vi "CreatePrivateEvents.vi"(8 "error in (no error)":errorcluster, 11 "SMO.Instrument":refnum<class "SMO.Instrument.lvclass">) -> (0 "error out":errorcluster, 3 "SMO.Instrument out":refnum<class "SMO.Instrument.lvclass">)   [LabVIEW 2019, in "SMO.Instrument.lvclass"]
doc: "JKI State Machine Objects (SMO) 1.1.0.20\nJKI - JKI\nCopyright (c) 2016, JKI"
uses:
  SMO.Instrument.lvclass
  SMO.Instrument.lvclass/SMO.Instrument.ctl
  Typedefs/API Inputs--Cluster.ctl
  Typedefs/Data.ctl
  vi.lib/JKI/JKI SMO/SMO/SMO.lvclass
panel:
  # "For instructions on how to use the JKI State Machine Objects, examples and video tutorials, visit:\nhttp://jki.net/state-machine-objects/\n\nJKI State Machine Objects™\nhttp://jki.net/state-machine-objects/\nCopyright (C) 2005-2015, JKI <info@jki.net>\nALL RIGHTS RESERVED"
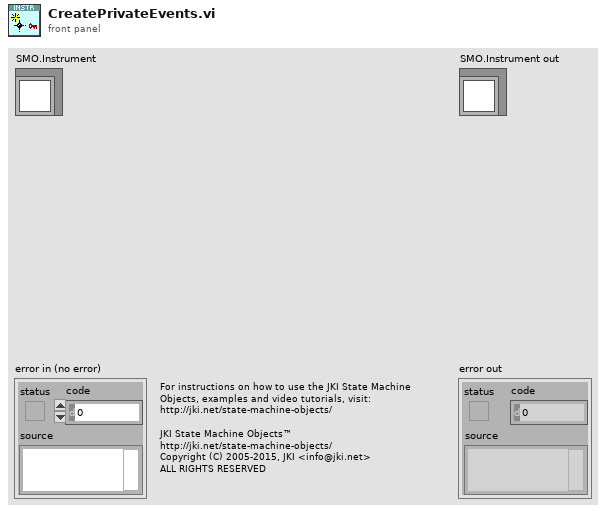
[diagram p1: front panel]
types:
  T1 = typedef "SMO.Instrument.lvclass/PrivateData--Ref.ctl" = refnum<data-value>
  T2 = typedef "SMO.Instrument.lvclass/API Inputs--Cluster.ctl" = cluster{"Data":T3}
  T3 = typedef "SMO.Instrument.lvclass/Data.ctl" = string
  T4 = typedef "SMO.Instrument.lvclass/PrivateData--Cluster.ctl" = cluster{"Configuration":T5, "Public Events":T6, "Protected Events":T7, "Private Events":T8, "Data":T3}
  T5 = typedef "SMO.Instrument.lvclass/Configuration--Cluster.ctl" = cluster{"Suffix":string}
  T6 = typedef "SMO.Instrument.lvclass/PublicEvents--Cluster.ctl" = cluster{"Data Changed":refnum<user-event>}
  T7 = typedef "SMO.Instrument.lvclass/ProtectedEvents--Cluster.ctl" = cluster{"API_Template":refnum<user-event>}
  T8 = typedef "SMO.Instrument.lvclass/PrivateEvents--Cluster.ctl" = cluster{"AsyncMethod":refnum<user-event>}
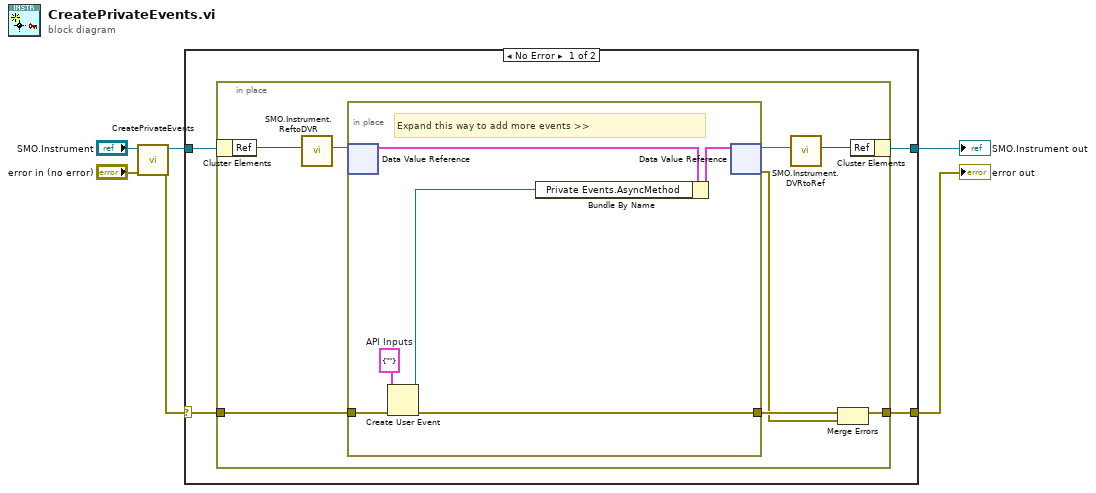
[diagram p0: block diagram]
diagram:
  n1 = call-parent "CreatePrivateEvents.vi"("error in (no error)"="error in (no error)", "SMO"="SMO.Instrument") -> ("error out"=w4:errorcluster, "SMO out"=w2:refnum<class "SMO.Instrument.lvclass">)  [unwired: 8 in]
  n2 = case shown="No Error" w4 {
    selector: w4 -> [w8 w26]
    tunnel: [w7 w26] -> w3
    tunnel: [w9 w25] -> w1
    tunnel: w2 -> [w10 w25]
    frame No Error {
      n3 = in-place {
        in-place-border: w8 -> [w18]
        in-place-border: [w15] -> w7
        n4 = in-place-cluster #1(w10) -> ("Ref"=w14:u32)
        n5 = call "SMO.Instrument.ReftoDVR.vi"("Ref"=w14) -> ("Ref"=w13:T1)  [unwired: 10 in]
        n6 = in-place {
          in-place-border: w18 -> [w22]
          in-place-border: [w23] -> w17
          w19 = T2 {"Data"=""}  # API Inputs
          # "Expand this way to add more events >>"
          n7 = in-place-dvr #2(w13) -> (w21:T4)  [unwired: 1 out]
          n8 = Create User Event(user event datatype=w19, error in=w22) -> (user event=w20:refnum<user-event>, error out=w23:errorcluster)
          n9 = Bundle By Name(cluster=w21, "Private Events.AsyncMethod"=w20) -> (w24:T4)
          n10 = in-place-dvr #2(w24) -> (w12:T1, w16:errorcluster)
        }
        n11 = call "SMO.Instrument.DVRtoRef.vi"("Ref"=w12) -> ("Ref"=w11:u32)  [unwired: 10 in]
        n12 = Merge Errors(w17, w16) -> (w15:errorcluster)
        n13 = in-place-cluster #1("Ref"=w11) -> (w9:refnum<class "SMO.Instrument.lvclass">)
      }
    }
    frame Error {
    }
  }
  "error out" <- w3
  "SMO.Instrument out" <- w1
